vi "Host - receiver.vi"() -> ()   [LabVIEW 2017]
panel:
  out "data out":string
  in  "stop":bool
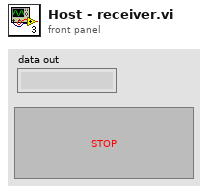
[diagram p1: front panel]
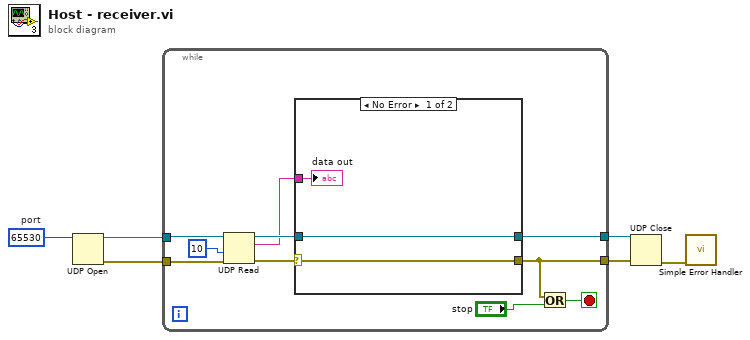
[diagram p0: block diagram]
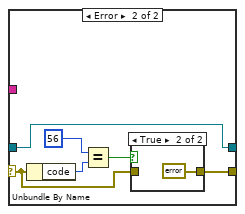
[diagram p2: hidden frame]
diagram:
  w4 = u16 65530  # port
  n1 = UDP Open(11:w4) -> (port=w6:refnum<k16>, 0:w5:errorcluster)  [unwired: 4 in, 1 out]
  n2 = while {
    tunnel: w6 -> [w16]
    tunnel: w5 -> [w15]
    tunnel: [w8] -> w3
    tunnel: [w10] -> w2
    stop <- w9 stop-if-true
    n3 = UDP Read(connection ID=w16, timeout ms (25000)=10, 8:w15) -> (data out=w11:string, error out=w13:errorcluster, 3:w12:refnum<k16>)  [unwired: 1 in, 2 out]
    n4 = case shown="No Error" w13 {
      selector: w13 -> [w19 w21]
      tunnel: w12 -> [w18 w20]
      tunnel: w11 -> [w17 _]
      tunnel: [w19 w22] -> w8
      tunnel: [w18 w20] -> w10
      frame No Error {
        "data out" <- w17
      }
      frame Error {
        n5 = Unbundle By Name(w21) -> ("code"=w25:i32)
        n6 = Equal?(x=56, y=w25) -> (x = y?=w23:bool)
        n7 = case shown="True" w23 {
          tunnel: [w26 errorcluster {"status"=FALSE, "code"=0, "source"=""} ("error constant")] -> w22
          tunnel: w21 -> [w26 _]
          frame False {
          }
          frame True {
          }
        }
      }
    }
    n8 = Or(x=w8, y="stop") -> (x .or. y?=w9:bool)
  }
  n9 = UDP Close(connection ID=w2, 8:w3) -> (error out=w1:errorcluster)  [unwired: 1 out]
  n10 = call <vilib>:"Simple Error Handler.vi"("error in (no error)"=w1) -> ()  [unwired: 4 in, 5 out]
